vi "Get Basic Mov wrapper.vi"(7 "bLoop":bool, 8 "error in (no error)":errorcluster caption="错误输入（无错误）", 10 "dwCanNodeId":u32, 11 "dwDevIndex":u32) -> (0 "error out":errorcluster caption="错误输出", 1 "pBasicMovObj out":cluster{"iSpd":i32, "iPos":i32, "iTimeOut":i32}, 3 "function return":u32)   [LabVIEW 2016, in "UISimCanFunc_wrapper.lvlib"]
doc: "_declspec (dllexport) DWORD GetBasicMov_wrapper(DWORD dwDevIndex, DWORD dwCanNodeId, P_BASIC_MOVE_PARA_OBJ pBasicMovObj, BOOL bLoop);"
uses:
  <userlib>/UISimCanFunc_wrapper/UISimCanFunc_wrapper.lvlib
  <userlib>/UISimCanFunc_wrapper/UISimCanFunc_wrapper.dll
panel:
  in  "pBasicMovObj":cluster{"iSpd":i32, "iPos":i32, "iTimeOut":i32}
  # "Works normally in both closed & open loops!\nWill ENABLE motor automatically."
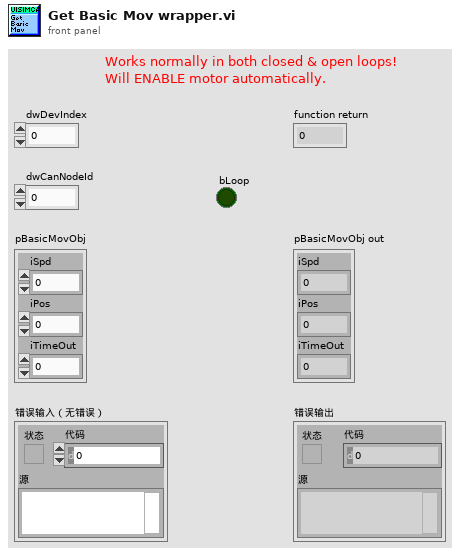
[diagram p1: front panel]
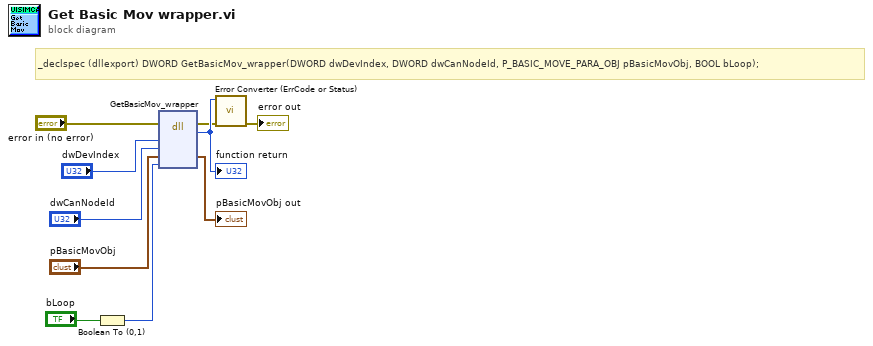
[diagram p0: block diagram]
diagram:
  # "_declspec (dllexport) DWORD GetBasicMov_wrapper(DWORD dwDevIndex, DWORD dwCanNodeId, P_BASIC_MOVE_PARA_OBJ pBasicMovObj, BOOL bLoop);"
  n1 = Boolean To (0,1)(Boolean="bLoop") -> (0, 1=w1:i16)
  n2 = dll-call lib="C:/Program Files (x86)/National Instruments/LabVIEW 2016/user.lib/UISimCanFunc_wrapper/UISimCanFunc_wrapper.*" fn="GetBasicMov_wrapper"(error in="error in (no error)", "dwDevIndex"="dwDevIndex", "dwCanNodeId"="dwCanNodeId", "pBasicMovObj"="pBasicMovObj", "bLoop"=w1) -> (error out=w4:errorcluster, w10:u32, "pBasicMovObj"=→"pBasicMovObj out":cluster{"iSpd":i32, "iPos":i32, "iTimeOut":i32})  [unwired: 5 in, 1 out]
  "function return" <- w10
  n3 = call <userlib>:"Error Converter (ErrCode or Status).vi"("error in (no error)"=w4, "error code"=w10) -> ("error out"=→"error out":errorcluster)  [unwired: 9 in]
